vi "LVClass_CorrectionDataManager dtor.vi"(0 "CorrectionDataManager in":refnum<class "CorrectionDataManager.lvclass">, 11 "error in (no error)":errorcluster) -> (4 "CorrectionDataManager out":refnum<class "CorrectionDataManager.lvclass">, 15 "error out":errorcluster)   [LabVIEW 2020, in "CorrectionDataManager.lvclass"]
doc: "CorrDataManager copy destructor.\n\n<B>corrdata_managerIn</B> : CorrDataManager object.\n<B>corrdata_managerOut</B> : CorrDataManager object."
uses:
  CorrectionDataManager.lvclass
  CorrectionDataManager.lvclass/CorrectionDataManager.ctl
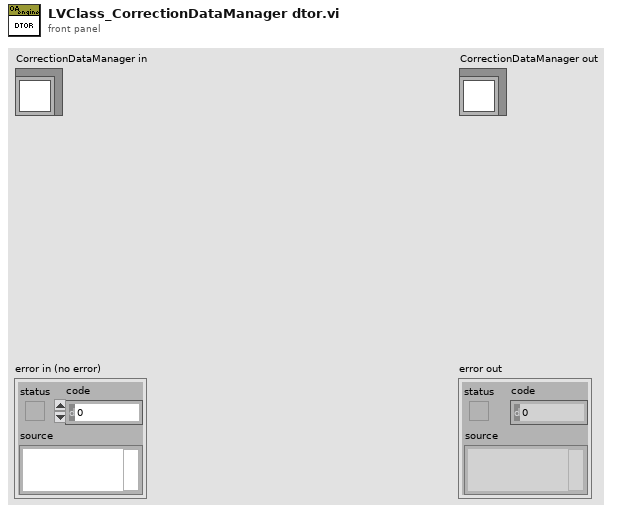
[diagram p1: front panel]
types:
  T1 = typedef "Handle creation.ctl" = enum16{"By ctor", "By write function"}
  T2 = typedef "ClassID.ctl" = i64
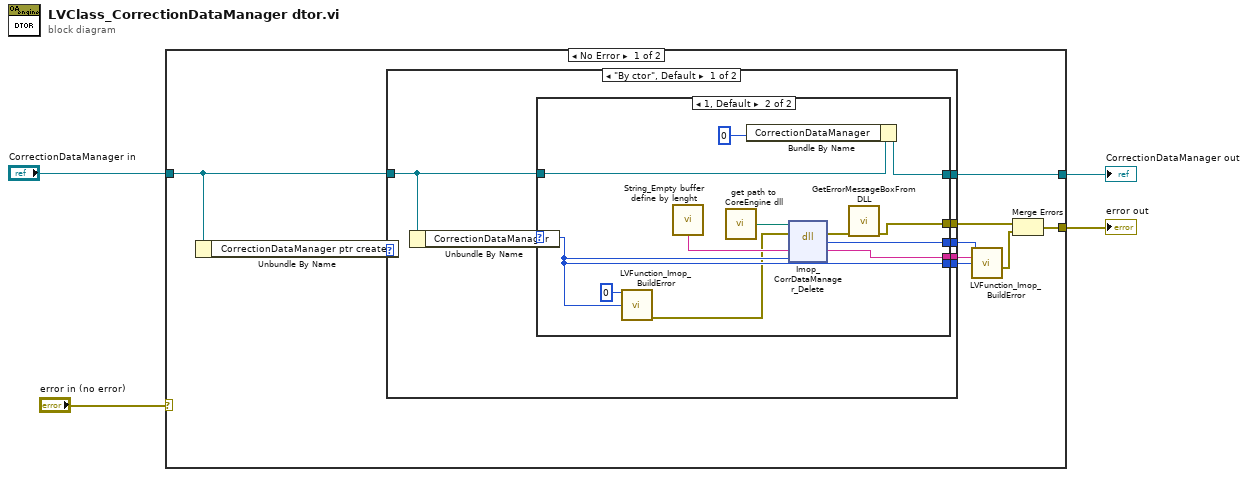
[diagram p0: block diagram]
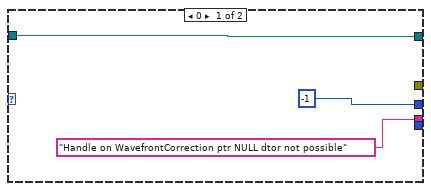
[diagram p2: hidden frame]
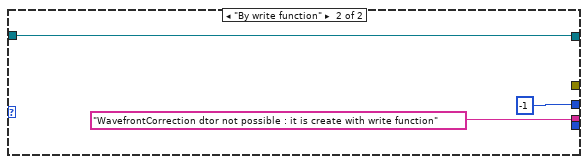
[diagram p3: hidden frame]
diagram:
  n1 = case shown="No Error" "error in (no error)" {
    selector: "error in (no error)" -> [_ w39]
    tunnel: "CorrectionDataManager in" -> [w10 w40]
    tunnel: [w11 w40] -> w2
    tunnel: [w6 w39] -> w1
    frame No Error {
      n2 = Unbundle By Name(w10) -> ("CorrectionDataManager ptr create"=w9:T1)
      n3 = case shown="\"By ctor\", Default" w9 {
        tunnel: [w20 "WavefrontCorrection dtor not possible : it is create with write function" ("message")] -> w13
        tunnel: [w19 -1] -> w12
        tunnel: w10 -> [w17 w36]
        tunnel: [w18 w36] -> w11
        tunnel: [w15 _] -> w8
        tunnel: [w14 _] -> w5
        frame "By ctor", Default {
          n4 = Unbundle By Name(w17) -> ("CorrectionDataManager"=w16:T2)
          n5 = case shown="1, Default" w16 {
            selector: w16 -> [_ w25]
            tunnel: ["Handle on WavefrontCorrection ptr NULL dtor not possible" ("message") w34] -> w20
            tunnel: [-1 w33] -> w19
            tunnel: w17 -> [w21 w29]
            tunnel: [w21 w28] -> w18
            tunnel: [_ w27] -> w15
            tunnel: [_ w25] -> w14
            frame 0 {
            }
            frame 1, Default {
              n6 = call "LVFunction_Imop_BuildError.vi"("code"=0, "Adresse"=w25) -> ("error out"=w24:errorcluster)  [unwired: 13 in]
              n7 = call "String_Empty buffer define by lenght.vi"() -> ("Empty buffer"=w35:string)  [unwired: 1 in]
              n8 = call "get path to CoreEngine dll.vi"() -> ("path to wavekit library"=w32:path)  [unwired: 14 in, 1 out]
              n9 = Bundle By Name(cluster=w29, "CorrectionDataManager"=u32 0 ("HasoEgine")) -> (w28:refnum<class "CorrectionDataManager.lvclass">)
              n10 = dll-call lib="D:/soft/HASO_v3/SVN_trunk/ImOpCoreEngine4_LV2011/DLLs/c_interface_vc100.dll" fn="Imop_CorrDataManager_Delete"(path in=w32, error in=w24, "message"=w35, "WavefrontCorrection"=w25) -> (error out=w31:errorcluster, "return type"=w33:i32, "message"=w34:string)  [unwired: 2 in, 1 out]
              n11 = call "GetErrorMessageBoxFromDLL.vi"("error IN"=w31) -> ("error OUT"=w27:errorcluster)  [unwired: 10 in]
            }
          }
        }
        frame "By write function" {
        }
      }
      n12 = call "LVFunction_Imop_BuildError.vi"("code"=w12, "String to Prepend to source (\"\")"=w13, "Adresse"=w5) -> ("error out"=w7:errorcluster)  [unwired: 12 in]
      n13 = Merge Errors(w8, w7) -> (w6:errorcluster)
    }
    frame Error {
    }
  }
  "error out" <- w1
  "CorrectionDataManager out" <- w2
